vi "Connection Monitor - Stop.vi"(8 "error in (no error)":errorcluster, 11 "RemoteControl.ZMQ in":refnum<class "RemoteControl.ZMQ.lvclass">) -> (0 "error out":errorcluster, 3 "RemoteControl.ZMQ out":refnum<class "RemoteControl.ZMQ.lvclass">)   [LabVIEW 2019, in "RemoteControl.ZMQ.lvclass"]
uses:
  RemoteControl.ZMQ.lvclass
  <vilib>/addons/zeromq/zmq_context.lvclass
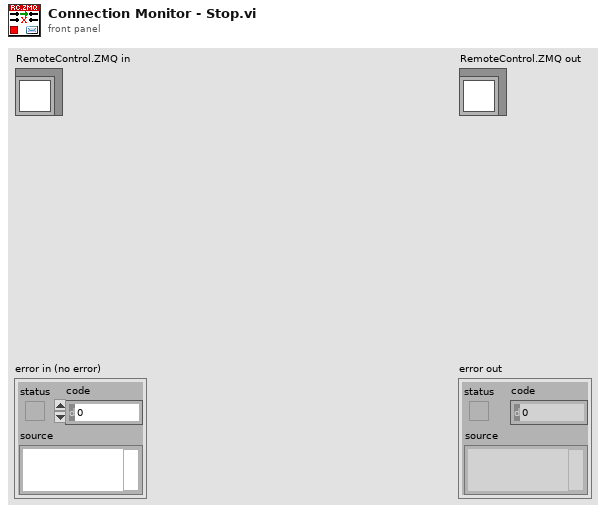
[diagram p1: front panel]
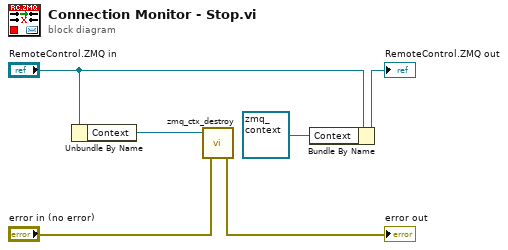
[diagram p0: block diagram]
diagram:
  n1 = Unbundle By Name("RemoteControl.ZMQ in") -> ("Context"=w6:refnum<class "zmq_context.lvclass">)
  n2 = call <vilib>:"zmq_ctx_destroy.vi"("error in"="error in (no error)", "context in"=w6) -> ("error out"=→"error out":errorcluster)  [unwired: 3 in]
  n3 = Bundle By Name(cluster="RemoteControl.ZMQ in", "Context"=refnum<class "zmq_context.lvclass"> refnum) -> (→"RemoteControl.ZMQ out":refnum<class "RemoteControl.ZMQ.lvclass">)
